vi "Mapping主程序.vi"() -> ()   [LabVIEW 2018]
uses:
  <vilib>/Instr/_visa.llb/VISA Configure Serial Port (Instr).vi
panel:
  in  "确认设置\nConfirm Setting":bool
  in  "扫描宽度Width of Rectangle(um)(X direction)":dbl format="%#g"
  in  "扫描长度Length of Rectangle(um)(Y direction)":dbl format="%#g"
  in  "Y 初始化值 Initial Value of Y (V2)":i64=32000
  in  "X 初始化值 Initial value of X (V1)":i64=32000
  out "当前X坐标 \nCurrent X":i64
  out "当前Y坐标\nCurrent Y":i64
  out "点间距(以步数计)":i64
  out "Y方向采点数量\nNum of Data Points \nin Y Direction":i64
  out "X方向采点数量\nNum of Data Points in X Direction":i64
  out "y方向总步数":i64
  out "x方向总步数":i64
  in  "采点间距 Distance Between Data Points(um)":dbl caption="采点间距(um)" format="%#g"
  out "宽度(X轴方向)\nWidth(X direction)":i32
  out "长度(y轴方向)\nLength(Y direction)":i32
  out "扫描起点y(将初始化点视为原点)":i64
  out "扫描起点x(将初始化点视为原点)":i64
  out "V2当前电压 V2_Voltage":dbl format="%_6g"
  out "V1当前电压 V1_Voltage":dbl format="%_6g"
  out "V2_Digital_Value":string
  out "V1_Digital_Value":string
  in  "启动扫描模式\nEnter Mapping Mode":bool
  in  "初始化 Initialize":bool
  in  "电压调节速度 Speed":u16(ring) items=["1", "2", "3"]
  in  "通道 Channel":u16(ring) items=["V1", "V2"]
  out "电压减少输出指示灯\nPilot Lamp of Reducing Voltage":bool
  in  "电压减少\nReduce Voltage":bool
  out "电压增加输出指示灯\nPilot Lamp of Increasing Voltage":bool
  in  "电压增加\nIncrease Voltage":bool
  in  "VISA resource name":refnum<visa-resource-name> caption="串口选项 Serial Port Option"
  in  "Stop":bool
  # "V"
  # "V"
  # "Note:\n1. The coordinate here is actually digital Value of Voltage in DAC\n, and on the camera the unit of coordinate  can be treated as ~0.05um\n2. \"Current X\" & \"Current Y\" is the coordinate relative to the initializing point\n(set by Initial value of X & Y)\n3. Current recommended initial value are: X=31855 Y=42495"
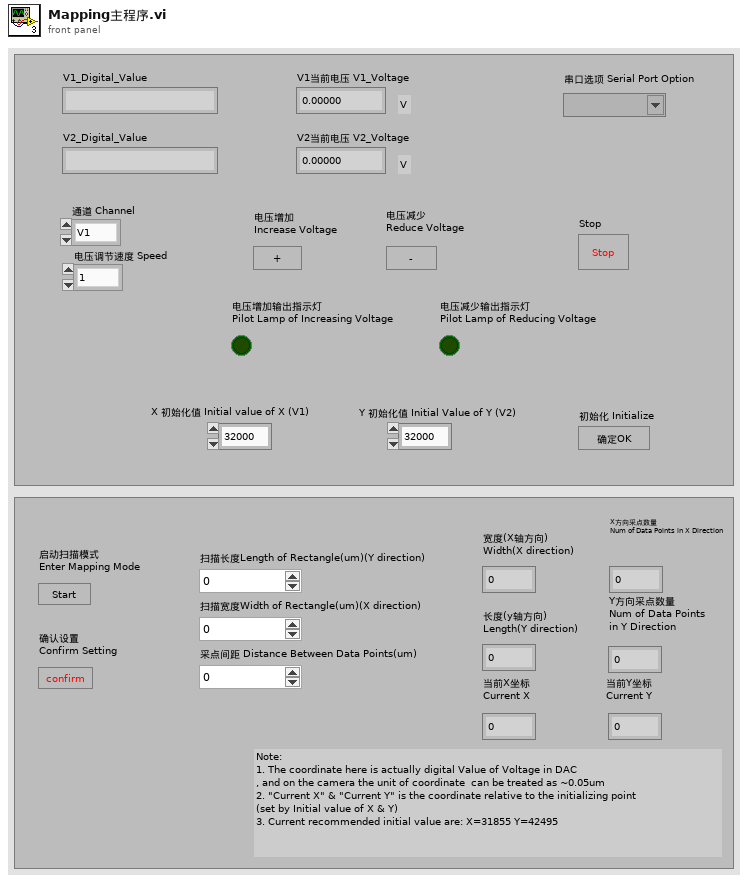
[diagram p1: front panel]
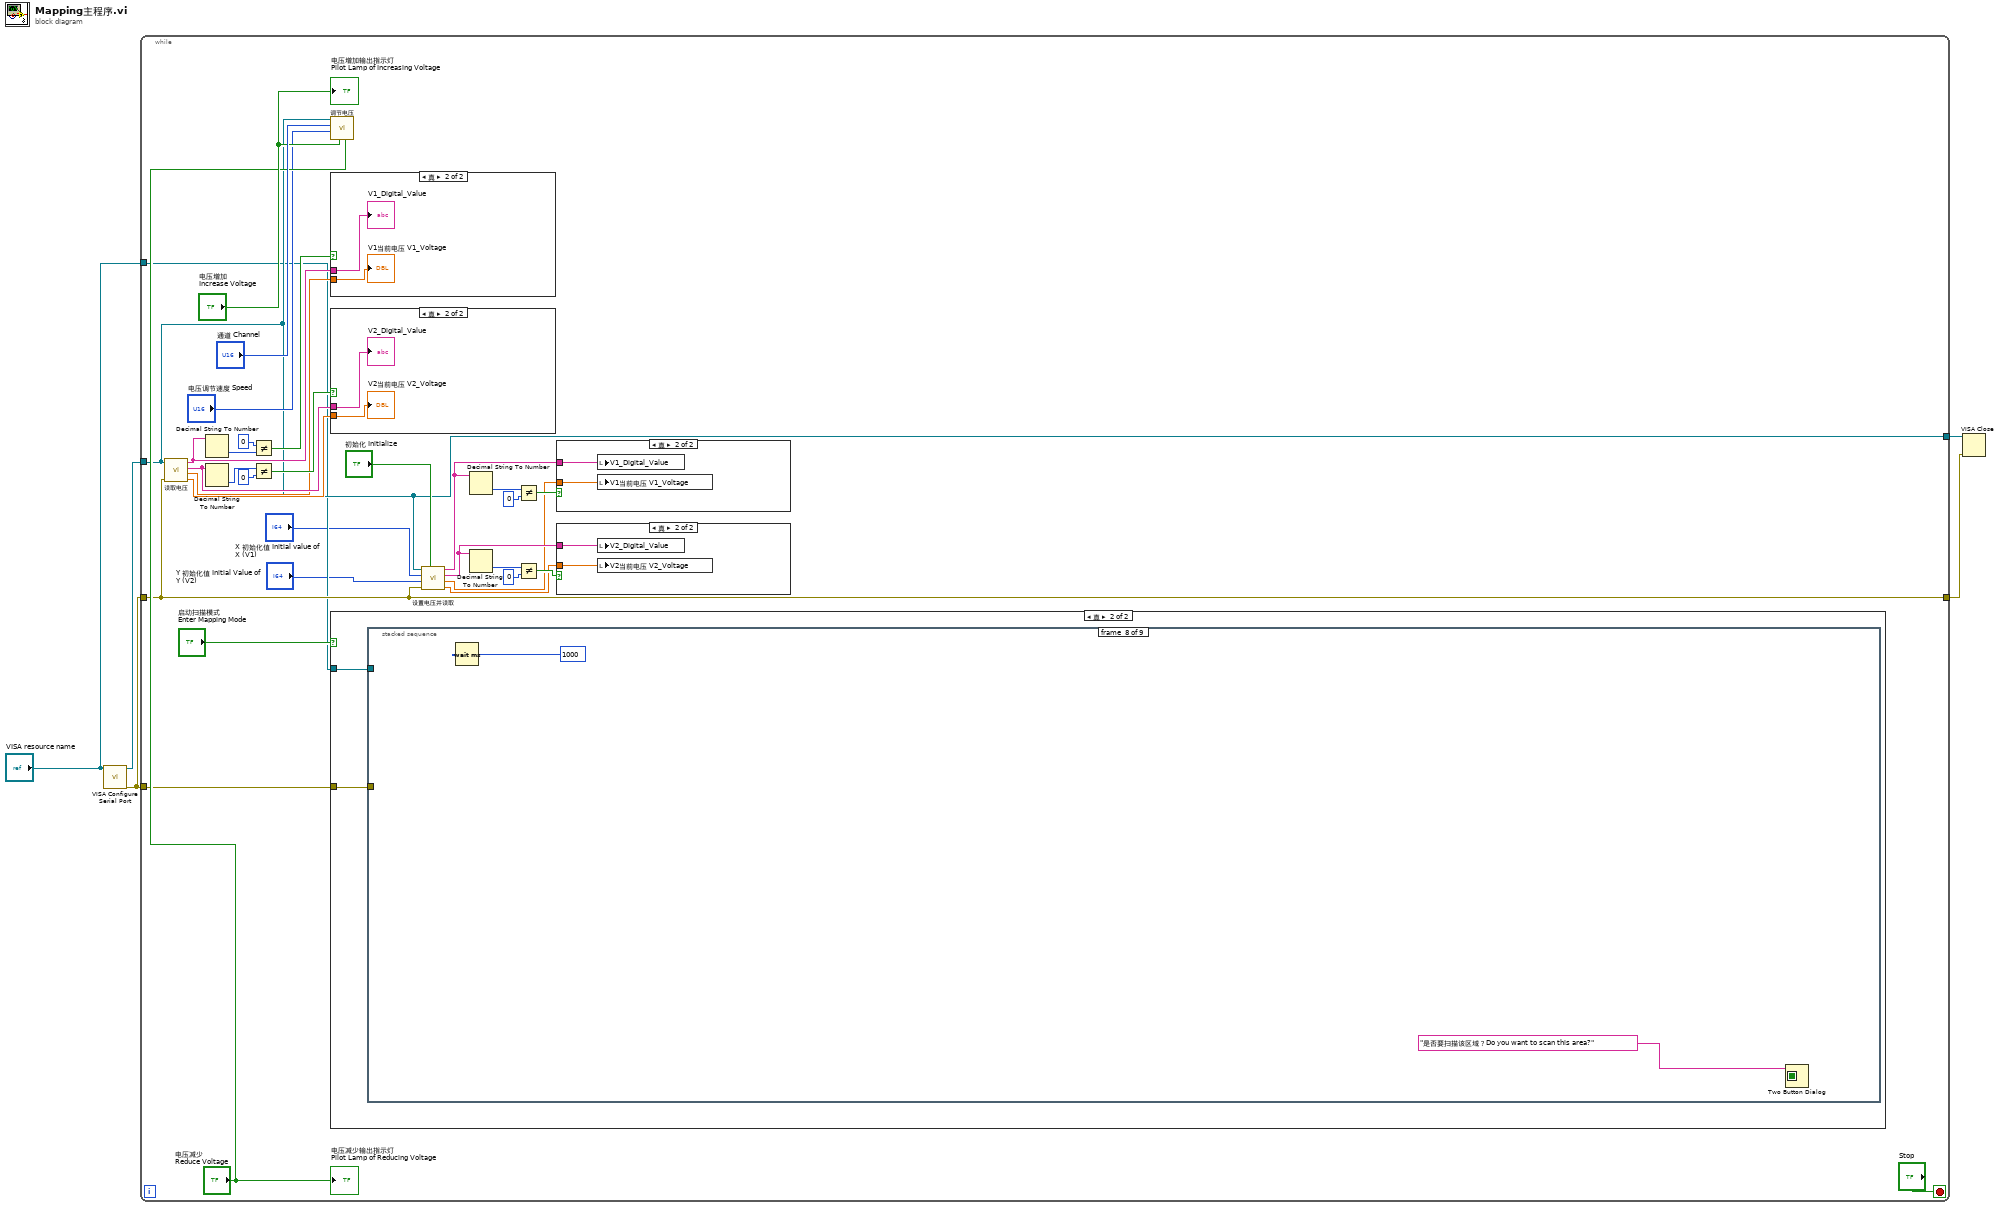
[diagram p0: block diagram]
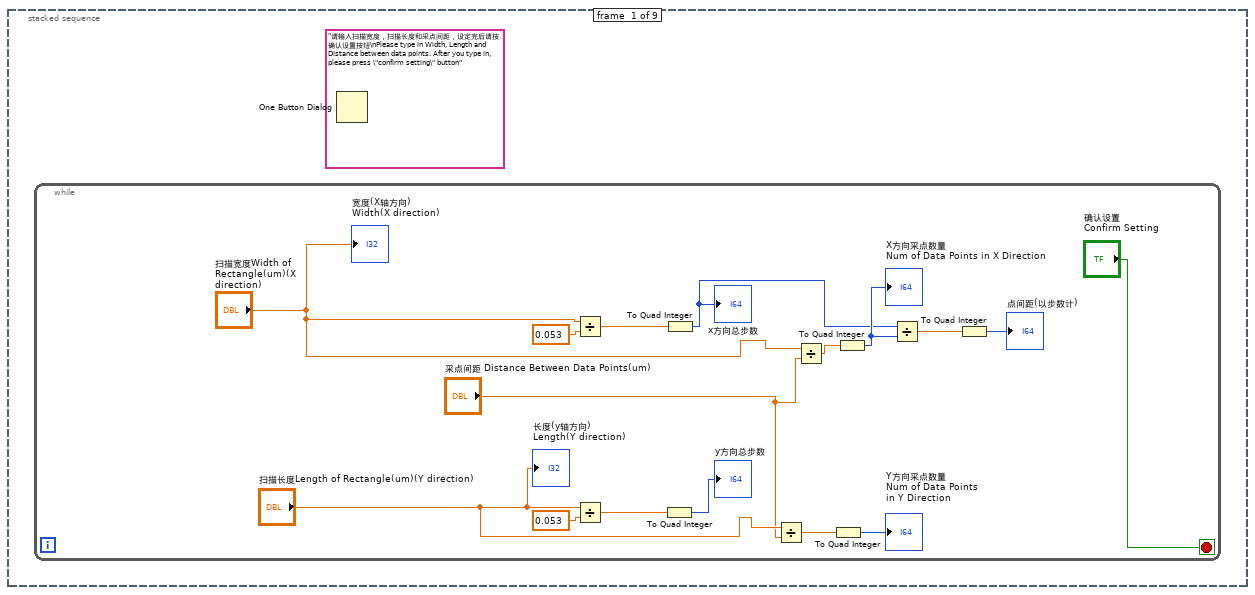
[diagram p3: hidden frame]
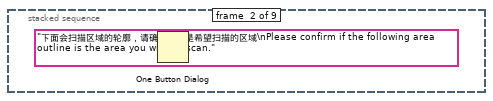
[diagram p4: hidden frame]
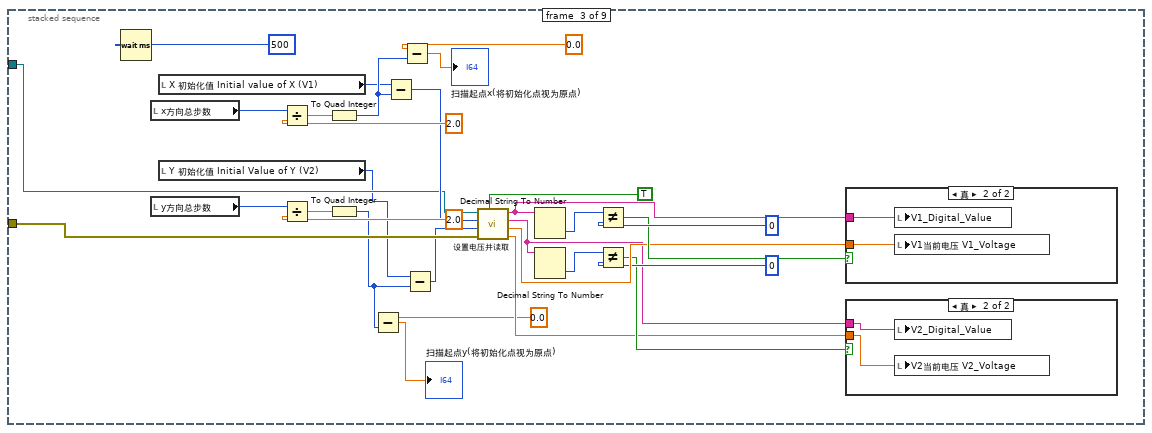
[diagram p5: hidden frame]
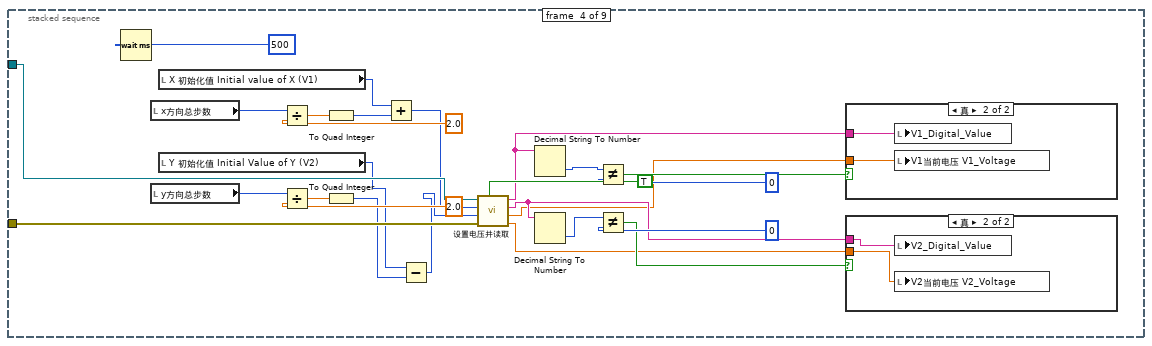
[diagram p8: hidden frame]
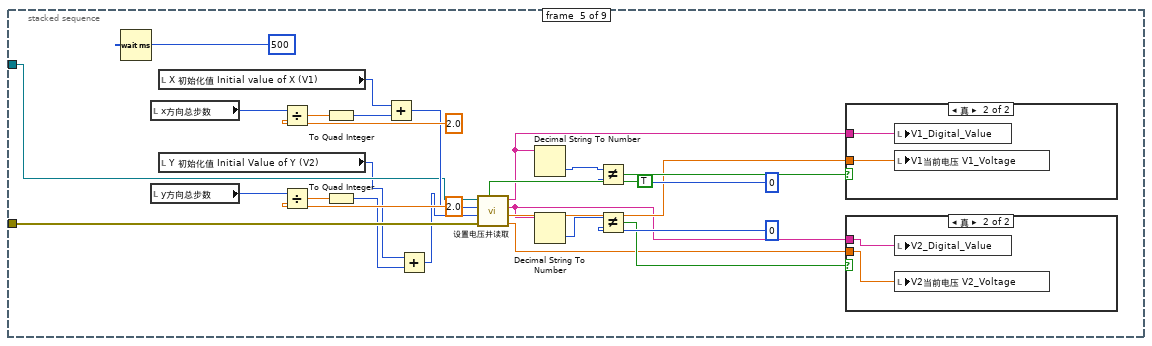
[diagram p11: hidden frame]
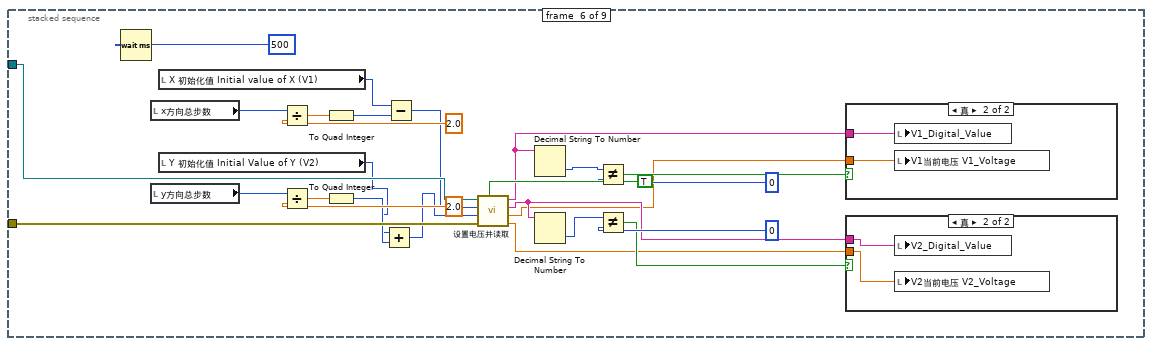
[diagram p14: hidden frame]
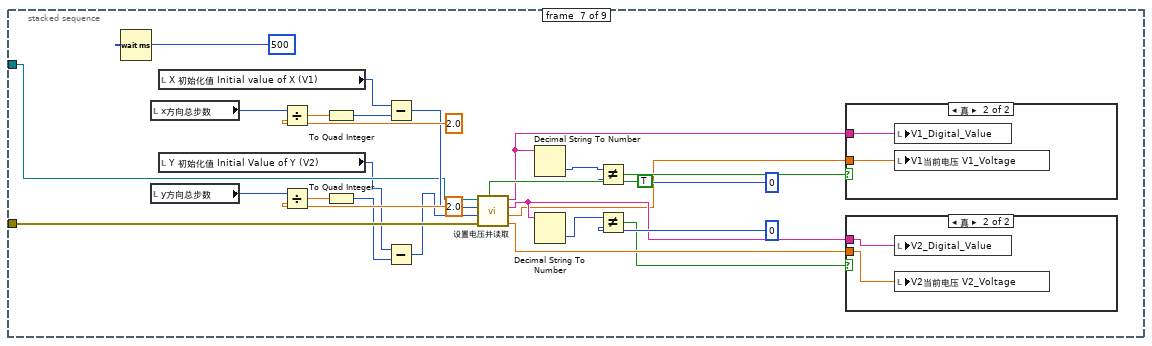
[diagram p17: hidden frame]
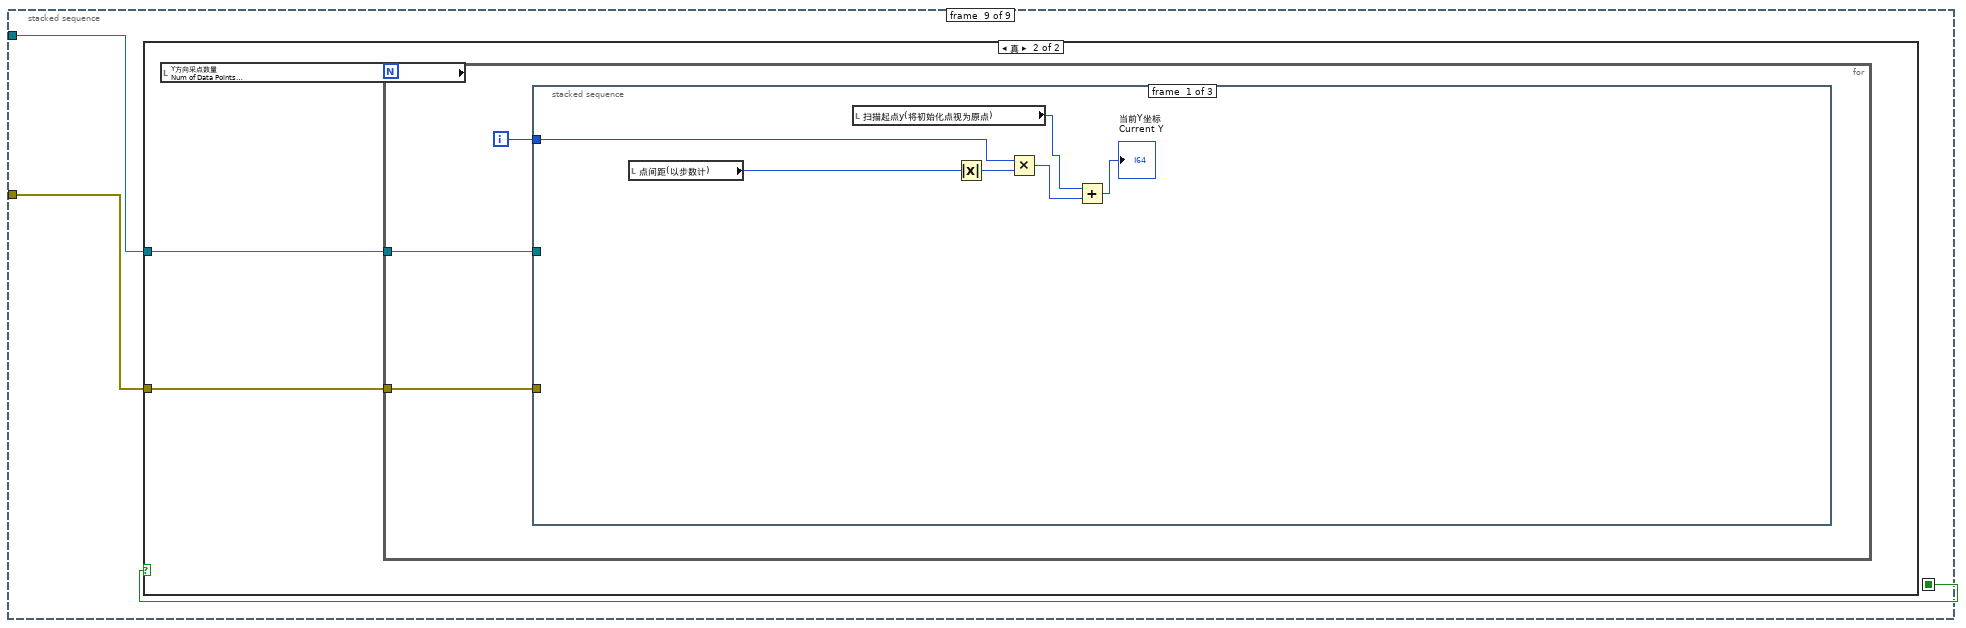
[diagram p20: hidden frame]
diagram:
  n1 = call-poly "VISA Configure Serial Port"("VISA resource name"="VISA resource name") -> ("VISA resource name out"=w5:refnum<visa-resource-name>, "error out"=w1:errorcluster)  [unwired: 13 in]
  n2 = while {
    tunnel: w1 -> [w23]
    tunnel: w5 -> [w21]
    tunnel: [w21] -> w4
    tunnel: [w23] -> w3
    tunnel: "VISA resource name" -> [w9]
    tunnel: w1 -> [w8]
    stop <- "Stop" stop-if-true
    n3 = call "读取电压.vi"("错误输入（无错误）"=w23, "VISA资源名称"=w21) -> ("V2当前电压"=w25:dbl, "V1当前电压"=w26:dbl, "V2_Digital"=w27:string, "V1_Digital"=w28:string)  [unwired: 6 in]
    n4 = Decimal String To Number(string=w28) -> (number=w34:i32)  [unwired: 2 in, 1 out]
    n5 = Decimal String To Number(string=w27) -> (number=w31:i32)  [unwired: 2 in, 1 out]
    n6 = Not Equal?(x=0, y=w34) -> (x != y?=w32:bool)
    n7 = Not Equal?(x=w31, y=0) -> (x != y?=w29:bool)
    n8 = call "调节电压.vi"("电压减少"="电压减少\nReduce Voltage", "电压增加"="电压增加\nIncrease Voltage", "电压调节速度"="电压调节速度 Speed", "通道 2"="通道 Channel", "引用"=w21) -> ()  [unwired: 5 in, 2 out]
    n9 = case shown="真" w32 {
      tunnel: w28 -> [_ w283]
      tunnel: w26 -> [_ w282]
      frame False {
      }
      frame True {
        "V1_Digital_Value" <- w283
        "V1当前电压 V1_Voltage" <- w282
      }
    }
    n10 = case shown="真" w29 {
      tunnel: w27 -> [_ w281]
      tunnel: w25 -> [_ w280]
      frame False {
      }
      frame True {
        "V2_Digital_Value" <- w281
        "V2当前电压 V2_Voltage" <- w280
      }
    }
    n11 = case shown="真" "启动扫描模式\nEnter Mapping Mode" {
      tunnel: w9 -> [_ w40]
      tunnel: w8 -> [_ w39]
      frame False {
      }
      frame True {
        n12 = stacked-sequence {
          seq-local: [_ _ _ _ _ _ _ w213 _] -> [_ _ _ _ _ _ _ _ w218]
          tunnel: w40 -> [_ _ w81 w112 w134 w168 w196 _ w217]
          tunnel: w39 -> [_ _ w80 w111 w133 w167 w195 _ w216]
          frame #0 {
            n13 = while {
              stop <- "确认设置\nConfirm Setting" stop-if-true
              n14 = Divide(x="扫描宽度Width of Rectangle(um)(X direction)", y=0.053) -> (x/y=w57:dbl)
              n15 = Divide(x="扫描长度Length of Rectangle(um)(Y direction)", y=0.053) -> (x/y=w55:dbl)
              n16 = To Quad Integer(1:w55) -> (0:→"y方向总步数":i64)
              n17 = To Quad Integer(1:w57) -> (0:w47:i64)
              "x方向总步数" <- w47
              n18 = Divide(x="扫描长度Length of Rectangle(um)(Y direction)", y="采点间距 Distance Between Data Points(um)") -> (x/y=w52:dbl)
              n19 = Divide(x="扫描宽度Width of Rectangle(um)(X direction)", y="采点间距 Distance Between Data Points(um)") -> (x/y=w53:dbl)
              n20 = To Quad Integer(1:w52) -> (0:→"Y方向采点数量\nNum of Data Points \nin Y Direction":i64)
              n21 = To Quad Integer(1:w53) -> (0:w50:i64)
              "X方向采点数量\nNum of Data Points in X Direction" <- w50
              n22 = Divide(x=w47, y=w50) -> (x/y=w49:dbl)
              n23 = To Quad Integer(1:w49) -> (0:→"点间距(以步数计)":i64)
              "长度(y轴方向)\nLength(Y direction)" <- "扫描长度Length of Rectangle(um)(Y direction)"
              "宽度(X轴方向)\nWidth(X direction)" <- "扫描宽度Width of Rectangle(um)(X direction)"
            }
            n24 = One Button Dialog(message="请输入扫描宽度，扫描长度和采点间距，设定完后请按确认设置按钮\nPlease type in Width, Length and Distance between data points. After you type in, please press \"confirm setting\" button" ("消息")) -> ()  [unwired: 1 in, 1 out]
          }
          frame #1 {
            n25 = One Button Dialog(message="下面会扫描区域的轮廓，请确认是否是希望扫描的区域\nPlease confirm if the following area outline is the area you wish to scan.") -> ()  [unwired: 1 in, 1 out]
          }
          frame #2 {
            n26 = Wait (ms)(milliseconds to wait=u32 500 ("等待时间（毫秒）")) -> ()  [unwired: 1 out]
            n27 = local read "x方向总步数"() -> (w79:i64)
            n28 = local read "y方向总步数"() -> (w78:i64)
            n29 = local read "X 初始化值 Initial value of X (V1)"() -> (w64:i64)
            n30 = local read "Y 初始化值 Initial Value of Y (V2)"() -> (w63:i64)
            n31 = Divide(x=w79, y=2.0) -> (x/y=w87:dbl)
            n32 = Divide(x=w78, y=2.0) -> (x/y=w85:dbl)
            n33 = To Quad Integer(1:w87) -> (0:w66:i64)
            n34 = To Quad Integer(1:w85) -> (0:w60:i64)
            n35 = Subtract(x=0.0, y=w60) -> (x-y=→"扫描起点y(将初始化点视为原点)":dbl)
            n36 = Subtract(x=w64, y=w66) -> (x-y=w83:i64)
            n37 = Subtract(x=0.0, y=w66) -> (x-y=→"扫描起点x(将初始化点视为原点)":dbl)
            n38 = Subtract(x=w63, y=w60) -> (x-y=w62:i64)
            n39 = call "设置电压并读取.vi"("布尔"=TRUE, "error out"=w80, "V2设置值"=w62, "V1设置值"=w83, "VISA resource name out"=w81) -> ("V2当前电压"=w68:dbl, "V1当前电压"=w73:dbl, "V2_Digital"=w69:string, "V1_Digital"=w74:string)  [unwired: 3 in]
            n40 = Decimal String To Number(string=w74) -> (number=w76:i32)  [unwired: 2 in, 1 out]
            n41 = Decimal String To Number(string=w69) -> (number=w71:i32)  [unwired: 2 in, 1 out]
            n42 = Not Equal?(x=w76, y=0) -> (x != y?=w75:bool)
            n43 = Not Equal?(x=w71, y=0) -> (x != y?=w70:bool)
            n44 = case shown="真" w75 {
              tunnel: w74 -> [_ w92]
              tunnel: w73 -> [_ w91]
              frame False {
              }
              frame True {
                n45 = local write "V1_Digital_Value"(w92) -> ()
                n46 = local write "V1当前电压 V1_Voltage"(w91) -> ()
              }
            }
            n47 = case shown="真" w70 {
              tunnel: w69 -> [_ w90]
              tunnel: w68 -> [_ w89]
              frame False {
              }
              frame True {
                n48 = local write "V2_Digital_Value"(w90) -> ()
                n49 = local write "V2当前电压 V2_Voltage"(w89) -> ()
              }
            }
          }
          frame #3 {
            n50 = Wait (ms)(milliseconds to wait=u32 500 ("等待时间（毫秒）")) -> ()  [unwired: 1 out]
            n51 = local read "x方向总步数"() -> (w108:i64)
            n52 = local read "y方向总步数"() -> (w107:i64)
            n53 = local read "X 初始化值 Initial value of X (V1)"() -> (w96:i64)
            n54 = local read "Y 初始化值 Initial Value of Y (V2)"() -> (w95:i64)
            n55 = Divide(x=w108, y=2.0) -> (x/y=w117:dbl)
            n56 = Divide(x=w107, y=2.0) -> (x/y=w115:dbl)
            n57 = To Quad Integer(1:w117) -> (0:w110:i64)
            n58 = To Quad Integer(1:w115) -> (0:w94:i64)
            n59 = Add(x=w96, y=w110) -> (x+y=w109:i64)
            n60 = Subtract(x=w95, y=w94) -> (x-y=w93:i64)
            n61 = call "设置电压并读取.vi"("布尔"=TRUE, "error out"=w111, "V2设置值"=w93, "V1设置值"=w109, "VISA resource name out"=w112) -> ("V2当前电压"=w97:dbl, "V1当前电压"=w98:dbl, "V2_Digital"=w99:string, "V1_Digital"=w100:string)  [unwired: 3 in]
            n62 = Decimal String To Number(string=w100) -> (number=w105:i32)  [unwired: 2 in, 1 out]
            n63 = Decimal String To Number(string=w99) -> (number=w103:i32)  [unwired: 2 in, 1 out]
            n64 = Not Equal?(x=w105, y=0) -> (x != y?=w102:bool)
            n65 = Not Equal?(x=w103, y=0) -> (x != y?=w101:bool)
            n66 = case shown="真" w102 {
              tunnel: w100 -> [_ w122]
              tunnel: w98 -> [_ w121]
              frame False {
              }
              frame True {
                n67 = local write "V1_Digital_Value"(w122) -> ()
                n68 = local write "V1当前电压 V1_Voltage"(w121) -> ()
              }
            }
            n69 = case shown="真" w101 {
              tunnel: w99 -> [_ w120]
              tunnel: w97 -> [_ w119]
              frame False {
              }
              frame True {
                n70 = local write "V2_Digital_Value"(w120) -> ()
                n71 = local write "V2当前电压 V2_Voltage"(w119) -> ()
              }
            }
          }
          frame #4 {
            n72 = Wait (ms)(milliseconds to wait=u32 500 ("等待时间（毫秒）")) -> ()  [unwired: 1 out]
            n73 = local read "x方向总步数"() -> (w136:i64)
            n74 = local read "y方向总步数"() -> (w135:i64)
            n75 = local read "X 初始化值 Initial value of X (V1)"() -> (w127:i64)
            n76 = local read "Y 初始化值 Initial Value of Y (V2)"() -> (w124:i64)
            n77 = Divide(x=w136, y=2.0) -> (x/y=w147:dbl)
            n78 = Divide(x=w135, y=2.0) -> (x/y=w145:dbl)
            n79 = To Quad Integer(1:w147) -> (0:w142:i64)
            n80 = To Quad Integer(1:w145) -> (0:w125:i64)
            n81 = Add(x=w127, y=w142) -> (x+y=w141:i64)
            n82 = Add(x=w124, y=w125) -> (x+y=w123:i64)
            n83 = call "设置电压并读取.vi"("布尔"=TRUE, "error out"=w133, "V2设置值"=w123, "V1设置值"=w141, "VISA resource name out"=w134) -> ("V2当前电压"=w128:dbl, "V1当前电压"=w130:dbl, "V2_Digital"=w126:string, "V1_Digital"=w129:string)  [unwired: 3 in]
            n84 = Decimal String To Number(string=w129) -> (number=w139:i32)  [unwired: 2 in, 1 out]
            n85 = Decimal String To Number(string=w126) -> (number=w137:i32)  [unwired: 2 in, 1 out]
            n86 = Not Equal?(x=w139, y=0) -> (x != y?=w132:bool)
            n87 = Not Equal?(x=w137, y=0) -> (x != y?=w131:bool)
            n88 = case shown="真" w132 {
              tunnel: w129 -> [_ w152]
              tunnel: w130 -> [_ w151]
              frame False {
              }
              frame True {
                n89 = local write "V1_Digital_Value"(w152) -> ()
                n90 = local write "V1当前电压 V1_Voltage"(w151) -> ()
              }
            }
            n91 = case shown="真" w131 {
              tunnel: w126 -> [_ w150]
              tunnel: w128 -> [_ w149]
              frame False {
              }
              frame True {
                n92 = local write "V2_Digital_Value"(w150) -> ()
                n93 = local write "V2当前电压 V2_Voltage"(w149) -> ()
              }
            }
          }
          frame #5 {
            n94 = Wait (ms)(milliseconds to wait=u32 500 ("等待时间（毫秒）")) -> ()  [unwired: 1 out]
            n95 = local read "x方向总步数"() -> (w166:i64)
            n96 = local read "y方向总步数"() -> (w165:i64)
            n97 = local read "X 初始化值 Initial value of X (V1)"() -> (w156:i64)
            n98 = local read "Y 初始化值 Initial Value of Y (V2)"() -> (w154:i64)
            n99 = Divide(x=w166, y=2.0) -> (x/y=w177:dbl)
            n100 = Divide(x=w165, y=2.0) -> (x/y=w175:dbl)
            n101 = To Quad Integer(1:w177) -> (0:w158:i64)
            n102 = To Quad Integer(1:w175) -> (0:w155:i64)
            n103 = Add(x=w154, y=w155) -> (x+y=w153:i64)
            n104 = Subtract(x=w156, y=w158) -> (x-y=w157:i64)
            n105 = call "设置电压并读取.vi"("布尔"=TRUE, "error out"=w167, "V2设置值"=w153, "V1设置值"=w157, "VISA resource name out"=w168) -> ("V2当前电压"=w159:dbl, "V1当前电压"=w160:dbl, "V2_Digital"=w161:string, "V1_Digital"=w163:string)  [unwired: 3 in]
            n106 = Decimal String To Number(string=w163) -> (number=w171:i32)  [unwired: 2 in, 1 out]
            n107 = Decimal String To Number(string=w161) -> (number=w169:i32)  [unwired: 2 in, 1 out]
            n108 = Not Equal?(x=w171, y=0) -> (x != y?=w164:bool)
            n109 = Not Equal?(x=w169, y=0) -> (x != y?=w162:bool)
            n110 = case shown="真" w164 {
              tunnel: w163 -> [_ w182]
              tunnel: w160 -> [_ w181]
              frame False {
              }
              frame True {
                n111 = local write "V1_Digital_Value"(w182) -> ()
                n112 = local write "V1当前电压 V1_Voltage"(w181) -> ()
              }
            }
            n113 = case shown="真" w162 {
              tunnel: w161 -> [_ w180]
              tunnel: w159 -> [_ w179]
              frame False {
              }
              frame True {
                n114 = local write "V2_Digital_Value"(w180) -> ()
                n115 = local write "V2当前电压 V2_Voltage"(w179) -> ()
              }
            }
          }
          frame #6 {
            n116 = Wait (ms)(milliseconds to wait=u32 500 ("等待时间（毫秒）")) -> ()  [unwired: 1 out]
            n117 = local read "x方向总步数"() -> (w194:i64)
            n118 = local read "y方向总步数"() -> (w193:i64)
            n119 = local read "X 初始化值 Initial value of X (V1)"() -> (w187:i64)
            n120 = local read "Y 初始化值 Initial Value of Y (V2)"() -> (w185:i64)
            n121 = Divide(x=w194, y=2.0) -> (x/y=w207:dbl)
            n122 = Divide(x=w193, y=2.0) -> (x/y=w204:dbl)
            n123 = To Quad Integer(1:w207) -> (0:w206:i64)
            n124 = To Quad Integer(1:w204) -> (0:w184:i64)
            n125 = Subtract(x=w187, y=w206) -> (x-y=w202:i64)
            n126 = Subtract(x=w185, y=w184) -> (x-y=w183:i64)
            n127 = call "设置电压并读取.vi"("布尔"=TRUE, "error out"=w195, "V2设置值"=w183, "V1设置值"=w202, "VISA resource name out"=w196) -> ("V2当前电压"=w188:dbl, "V1当前电压"=w189:dbl, "V2_Digital"=w190:string, "V1_Digital"=w191:string)  [unwired: 3 in]
            n128 = Decimal String To Number(string=w191) -> (number=w199:i32)  [unwired: 2 in, 1 out]
            n129 = Decimal String To Number(string=w190) -> (number=w197:i32)  [unwired: 2 in, 1 out]
            n130 = Not Equal?(x=w199, y=0) -> (x != y?=w192:bool)
            n131 = Not Equal?(x=w197, y=0) -> (x != y?=w186:bool)
            n132 = case shown="真" w192 {
              tunnel: w191 -> [_ w212]
              tunnel: w189 -> [_ w211]
              frame False {
              }
              frame True {
                n133 = local write "V1_Digital_Value"(w212) -> ()
                n134 = local write "V1当前电压 V1_Voltage"(w211) -> ()
              }
            }
            n135 = case shown="真" w186 {
              tunnel: w190 -> [_ w210]
              tunnel: w188 -> [_ w209]
              frame False {
              }
              frame True {
                n136 = local write "V2_Digital_Value"(w210) -> ()
                n137 = local write "V2当前电压 V2_Voltage"(w209) -> ()
              }
            }
          }
          frame #7 {
            n138 = Wait (ms)(milliseconds to wait=u32 1000 ("等待时间（毫秒）")) -> ()  [unwired: 1 out]
            n139 = Two Button Dialog(message="是否要扫描该区域？Do you want to scan this area?") -> (T button?=w213:bool)  [unwired: 2 in]
          }
          frame #8 {
            n140 = case shown="真" w218 {
              tunnel: w217 -> [_ w220]
              tunnel: w216 -> [_ w219]
              frame False {
              }
              frame True {
                n141 = local read "Y方向采点数量\nNum of Data Points \nin Y Direction"() -> (w221:i64)
                n142 = for {
                  N: w221 -> [_]
                  tunnel: w220 -> [w224]
                  tunnel: w219 -> [w223]
                  i -> [w222]
                  n143 = stacked-sequence {
                    tunnel: w222 -> [w230 _ _]
                    tunnel: w224 -> [_ w232 _]
                    tunnel: w223 -> [_ w231 _]
                    frame #0 {
                      n144 = local read "点间距(以步数计)"() -> (w229:i64)
                      n145 = local read "扫描起点y(将初始化点视为原点)"() -> (w227:i64)
                      n146 = Absolute Value(x=w229) -> (abs(x)=w228:i64)
                      n147 = Multiply(x=w230, y=w228) -> (x*y=w226:i64)
                      n148 = Add(x=w227, y=w226) -> (x+y=→"当前Y坐标\nCurrent Y":i64)
                    }
                    frame #1 {
                      n149 = local read "X方向采点数量\nNum of Data Points in X Direction"() -> (w233:i64)
                      n150 = for {
                        N: w233 -> [_]
                        tunnel: w232 -> [w239]
                        tunnel: w231 -> [w238]
                        i -> [w234]
                        n151 = flat-sequence {
                          tunnel: w238 -> [w245]
                          tunnel: w239 -> [w246]
                          tunnel: [w246] -> w236
                          tunnel: [w245] -> w235
                          tunnel: w234 -> [w241]
                          tunnel: w236 -> [w260]
                          tunnel: w235 -> [w259]
                          frame #0 {
                            n152 = local read "扫描起点x(将初始化点视为原点)"() -> (w242:i64)
                            n153 = local read "点间距(以步数计)"() -> (w240:i64)
                            n154 = Multiply(x=w241, y=w240) -> (x*y=w243:i64)
                            n155 = Add(x=w242, y=w243) -> (x+y=→"当前X坐标 \nCurrent X":i64)
                          }
                          frame #1 {
                            n156 = local read "Y 初始化值 Initial Value of Y (V2)"() -> (w248:i64)
                            n157 = local read "X 初始化值 Initial value of X (V1)"() -> (w251:i64)
                            n158 = local read "当前Y坐标\nCurrent Y"() -> (w249:i64)
                            n159 = local read "当前X坐标 \nCurrent X"() -> (w252:i64)
                            n160 = Add(x=w252, y=w251) -> (x+y=w250:i64)
                            n161 = Add(x=w249, y=w248) -> (x+y=w247:i64)
                            n162 = call "设置电压并读取.vi"("布尔"=TRUE, "error out"=w259, "V2设置值"=w247, "V1设置值"=w250, "VISA resource name out"=w260) -> ("V2当前电压"=w253:dbl, "V1当前电压"=w254:dbl, "V2_Digital"=w255:string, "V1_Digital"=w256:string)  [unwired: 3 in]
                            n163 = Decimal String To Number(string=w256) -> (number=w264:i32)  [unwired: 2 in, 1 out]
                            n164 = Decimal String To Number(string=w255) -> (number=w265:i32)  [unwired: 2 in, 1 out]
                            n165 = Not Equal?(x=w264, y=0) -> (x != y?=w258:bool)
                            n166 = Not Equal?(x=w265, y=0) -> (x != y?=w257:bool)
                            n167 = case shown="真" w258 {
                              tunnel: w256 -> [_ w269]
                              tunnel: w254 -> [_ w268]
                              frame False {
                              }
                              frame True {
                                n168 = local write "V1_Digital_Value"(w269) -> ()
                                n169 = local write "V1当前电压 V1_Voltage"(w268) -> ()
                              }
                            }
                            n170 = case shown="真" w257 {
                              tunnel: w255 -> [_ w267]
                              tunnel: w253 -> [_ w266]
                              frame False {
                              }
                              frame True {
                                n171 = local write "V2_Digital_Value"(w267) -> ()
                                n172 = local write "V2当前电压 V2_Voltage"(w266) -> ()
                              }
                            }
                          }
                        }
                        n173 = Wait (ms)(milliseconds to wait=u32 100 ("等待时间（毫秒）")) -> ()  [unwired: 1 out]
                      }
                    }
                    frame #2 {
                      n174 = local read "点间距(以步数计)"() -> (w271:i64)
                      n175 = local read "扫描起点x(将初始化点视为原点)"() -> (w275:i64)
                      n176 = Multiply(x=w271, y=i64 -1) -> (x*y=w270:i64)
                      n177 = local write "点间距(以步数计)"(w270) -> ()
                      n178 = Multiply(x=w275, y=i64 -1) -> (x*y=w273:i64)
                      n179 = local write "扫描起点x(将初始化点视为原点)"(w273) -> ()
                    }
                  }
                }
              }
            }
          }
        }
      }
    }
    n180 = call "设置电压并读取.vi"("布尔"="初始化 Initialize", "error out"=w23, "V2设置值"="Y 初始化值 Initial Value of Y (V2)", "V1设置值"="X 初始化值 Initial value of X (V1)", "VISA resource name out"=w21) -> ("V2当前电压"=w11:dbl, "V1当前电压"=w12:dbl, "V2_Digital"=w13:string, "V1_Digital"=w17:string)  [unwired: 3 in]
    n181 = Decimal String To Number(string=w17) -> (number=w19:i32)  [unwired: 2 in, 1 out]
    n182 = Decimal String To Number(string=w13) -> (number=w15:i32)  [unwired: 2 in, 1 out]
    n183 = Not Equal?(x=w19, y=0) -> (x != y?=w18:bool)
    n184 = Not Equal?(x=w15, y=0) -> (x != y?=w14:bool)
    n185 = case shown="真" w18 {
      tunnel: w17 -> [_ w279]
      tunnel: w12 -> [_ w278]
      frame False {
      }
      frame True {
        n186 = local write "V1_Digital_Value"(w279) -> ()
        n187 = local write "V1当前电压 V1_Voltage"(w278) -> ()
      }
    }
    n188 = case shown="真" w14 {
      tunnel: w13 -> [_ w277]
      tunnel: w11 -> [_ w276]
      frame False {
      }
      frame True {
        n189 = local write "V2_Digital_Value"(w277) -> ()
        n190 = local write "V2当前电压 V2_Voltage"(w276) -> ()
      }
    }
    "电压增加输出指示灯\nPilot Lamp of Increasing Voltage" <- "电压增加\nIncrease Voltage"
    "电压减少输出指示灯\nPilot Lamp of Reducing Voltage" <- "电压减少\nReduce Voltage"
  }
  n191 = VISA Close(VISA resource name=w4, error in (no error)=w3) -> ()  [unwired: 1 out]
